vi "HV_SWVMaxSet.vi"(10 "Max Voltage":string) -> (3 "standard output":string)   [LabVIEW 2018]
panel:
  # "- Set maximum software voltage to limit the voltage sent to the channels\n- Keep below 6000V for CAEN V6534 HV card"
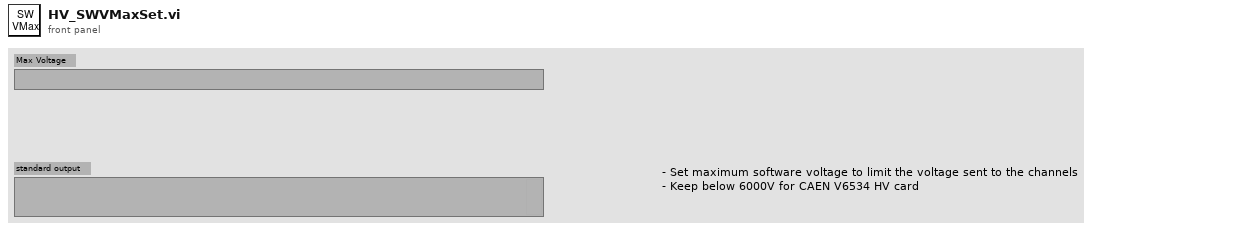
[diagram p1: front panel]
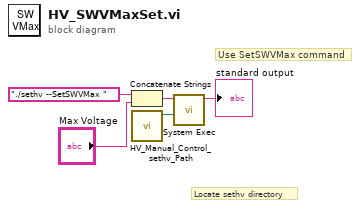
[diagram p0: block diagram]
diagram:
  # "Locate sethv directory"
  # "Use SetSWVMax command"
  n1 = Concatenate Strings("./sethv --SetSWVMax " ("string"), "Max Voltage") -> (w3:string)
  n2 = call "HV_Manual_Control_sethv_Path.vi"() -> ("sethv filepath"=w1:path)  [unwired: 11 in]
  n3 = call <vilib>:"System Exec.vi"("working directory"=w1, "command line"=w3) -> ("standard output"=→"standard output":string)  [unwired: 6 in, 3 out]
